vi "conditional_error_clearer.vi"(7 "clear?":bool=TRUE, 8 "error in (no error)":errorcluster, 10 "array of clearable error codes":i32[](array[numeric])) -> (0 "error out":errorcluster)   [LabVIEW 2010]
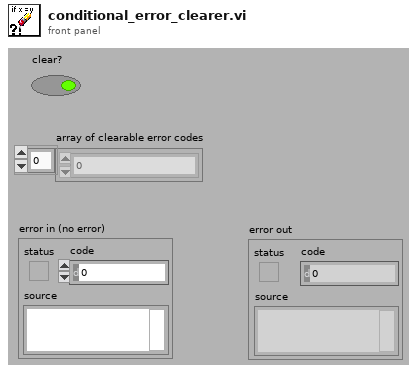
[diagram p1: front panel]
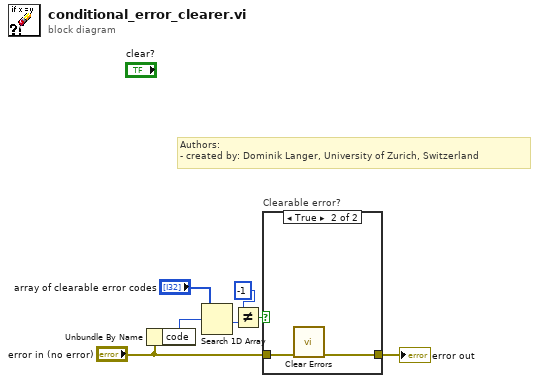
[diagram p0: block diagram]
diagram:
  # "Authors: \n- created by: Dominik Langer, University of Zurich, Switzerland"
  n1 = Unbundle By Name("error in (no error)") -> ("code"=w6:i32)
  n2 = Search 1D Array(1D array="array of clearable error codes", element=w6) -> (index of element=w3:i32)  [unwired: 1 out]
  n3 = Not Equal?(x=-1, y=w3) -> (x != y?=w2:bool)
  n4 = case "Clearable error?" shown="True" w2 {
    tunnel: "error in (no error)" -> [w8 w10]
    tunnel: [w8 w9] -> w4
    frame False {
    }
    frame True {
      n5 = call <vilib>:"Clear Errors.vi"("error in (no error)"=w10) -> ("error out"=w9:errorcluster)  [unwired: 6 out]
    }
  }
  "error out" <- w4
